vi "Liblinear - Split Problem.vi"(8 "error in (no error)":errorcluster, 9 "Seed (-1)":i32=-1, 10 "Validation fraction":dbl=0.2 caption="Validation fraction (0.2)" format="%#_13g", 11 "liblinear_problem":T1={"y"=[], "x"=[], "bias"=-1.0}) -> (0 "error out":errorcluster, 1 "Validation indices":i32[](array[numeric]), 2 "Validation set":T1={"y"=[], "x"=[], "bias"=-1.0}, 3 "Training set":T1={"y"=[], "x"=[], "bias"=-1.0}, 5 "Training indices":i32[](array[numeric]))   [LabVIEW 2015]
doc: "Splits the problem into a validation and training set, taking the amount of samples per class into account."
uses:
  Liblinear/Controls/liblinear_problem.ctl
  LibSVM Sparse/Wrapper API/Controls/svm_node.ctl
  <vilib>/Analysis/1siggen.llb/Riffle Array (I32).vi
  <vilib>/Analysis/NI_AALBase.lvlib
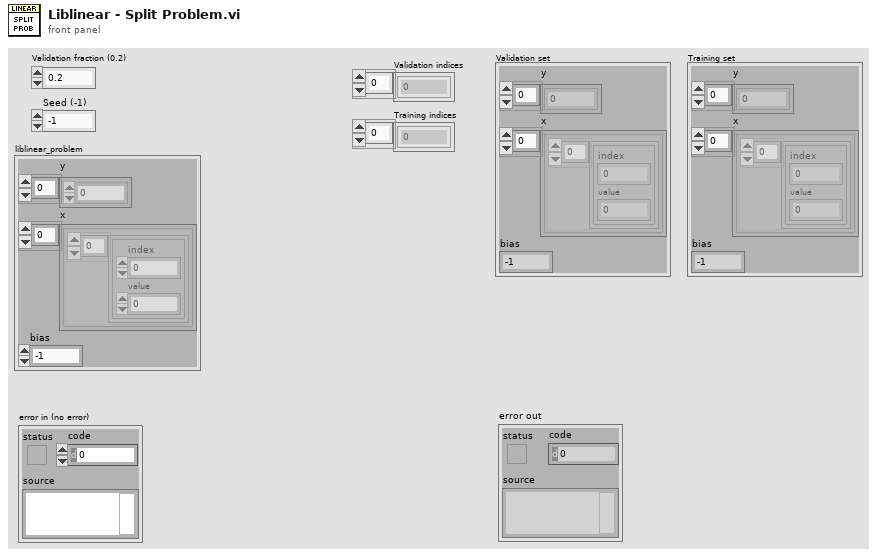
[diagram p1: front panel]
types:
  T1 = typedef "liblinear_problem.ctl" = cluster{"y":dbl[], "x":cluster{T2[]}[], "bias":dbl}
  T2 = typedef "svm_node.ctl" = cluster{"index":i32, "value":dbl}
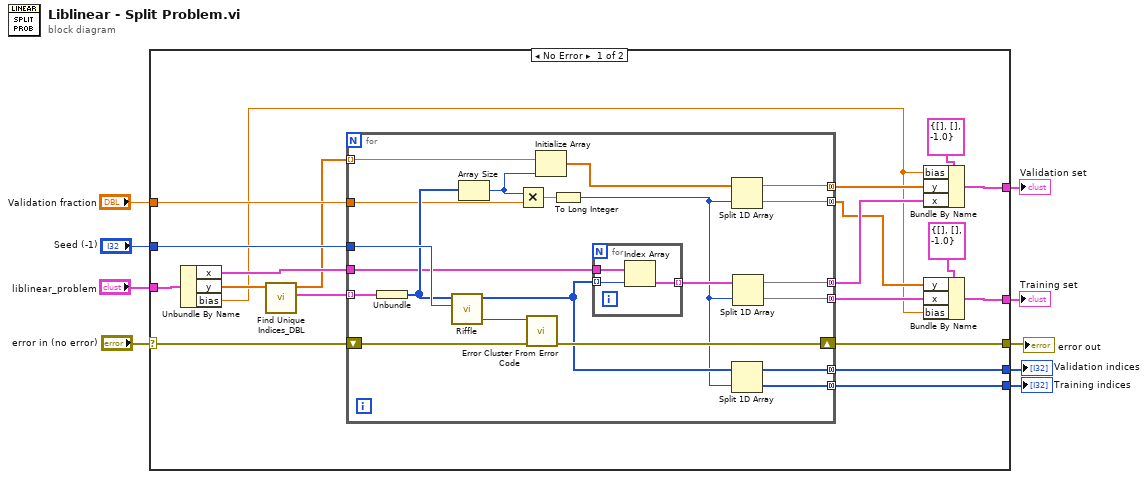
[diagram p0: block diagram]
diagram:
  n1 = case shown="No Error" "error in (no error)" {
    selector: "error in (no error)" -> [w25 w54]
    tunnel: [w17 w54] -> w9
    tunnel: "liblinear_problem" -> [w29 _]
    tunnel: "Seed (-1)" -> [w26 _]
    tunnel: "Validation fraction" -> [w23 _]
    tunnel: [w16 _] -> w1
    tunnel: [w15 _] -> w2
    tunnel: [w14 _] -> w5
    tunnel: [w13 _] -> w4
    frame No Error {
      n2 = Unbundle By Name(w29) -> ("x"=w24:cluster{T2[]}[], "y"=w28:dbl[], "bias"=w10:dbl)
      n3 = call "Find Unique Indices_DBL.vi"("Input Array"=w28) -> ("Unique indices"=w27:cluster{i32[]}[], "Unique values"=w22:dbl[])  [unwired: 9 in]
      n4 = for {
        tunnel: w27 -> [w50] mode=indexing
        tunnel: w26 -> [w49]
        shift-right: [w48] -> w17
        shift-left: w25 -> [w47]
        tunnel: w24 -> [w44]
        tunnel: w23 -> [w32]
        tunnel: [w42] -> w20 mode=concatenating
        tunnel: [w41] -> w18 mode=concatenating
        tunnel: w22 -> [w40] mode=indexing
        tunnel: [w38] -> w21 mode=concatenating
        tunnel: [w37] -> w19 mode=concatenating
        tunnel: [w35] -> w14 mode=concatenating
        tunnel: [w34] -> w13 mode=concatenating
        n5 = Unbundle(w50) -> (w45:i32[])
        n6 = call-poly <vilib>:"Riffle.vi"("seed"=w49, "X"=w45) -> ("error"=w46:i32, "Riffled {X}"=w36:i32[])  [unwired: 7 in, 1 out]
        n7 = Array Size(array=w45) -> (size(s)=w33:i32)
        n8 = Multiply(x=w33, y=w32) -> (x*y=w31:dbl)
        n9 = call <vilib>:"Error Cluster From Error Code.vi"("error in (no error)"=w47, "error code (0)"=w46) -> ("error out"=w48:errorcluster)  [unwired: 7 in]
        n10 = Initialize Array(w40, w33) -> (w39:dbl[])
        n11 = To Long Integer(number=w31) -> (32bit integer=w30:i32)
        n12 = for {
          tunnel: w36 -> [w52] mode=indexing
          tunnel: w44 -> [w53]
          tunnel: [w51] -> w43 mode=indexing
          n13 = Index Array(array=w53, index=w52) -> (element=w51:cluster{T2[]})
        }
        n14 = Split 1D Array(array=w39, index=w30) -> (first subarray=w38:dbl[], second subarray=w37:dbl[])
        n15 = Split 1D Array(array=w36, index=w30) -> (first subarray=w35:i32[], second subarray=w34:i32[])
        n16 = Split 1D Array(array=w43, index=w30) -> (first subarray=w42:cluster{T2[]}[], second subarray=w41:cluster{T2[]}[])
      }
      n17 = Bundle By Name(cluster=T1 {"y"=[], "x"=[], "bias"=-1.0} ("liblinear_problem"), "bias"=w10, "y"=w21, "x"=w20) -> (w15:T1)
      n18 = Bundle By Name(cluster=T1 {"y"=[], "x"=[], "bias"=-1.0} ("liblinear_problem"), "y"=w19, "x"=w18, "bias"=w10) -> (w16:T1)
    }
    frame Error {
    }
  }
  "error out" <- w9
  "Validation indices" <- w5
  "Training indices" <- w4
  "Validation set" <- w2
  "Training set" <- w1
